vi "NextToken.vi"(8 "error in (no error)":errorcluster, 10 "Index In":i32, 11 "JSON String":string) -> (0 "error out":errorcluster, 1 "TOKEN":T1, 2 "Index Out":i32)   [LabVIEW 2016, in "JSON Value.lvclass"]
uses:
  JSON Value.lvclass
  Token Type.ctl
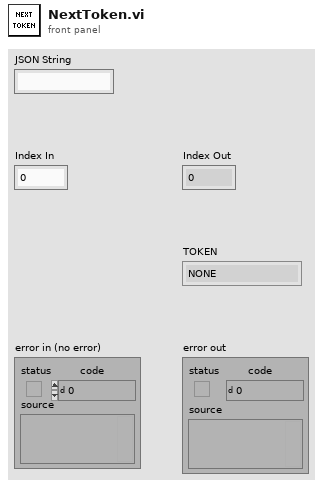
[diagram p1: front panel]
types:
  T1 = typedef "JSON Value.lvclass/Token Type.ctl" = enum8{"NONE", "CURLY_OPEN", "CURLY_CLOSE", "SQUARED_OPEN", "SQUARED_CLOSE", "COLON", "COMMA", "STRING", "NUMBER", "TRUE", "FALSE", "NULL"}
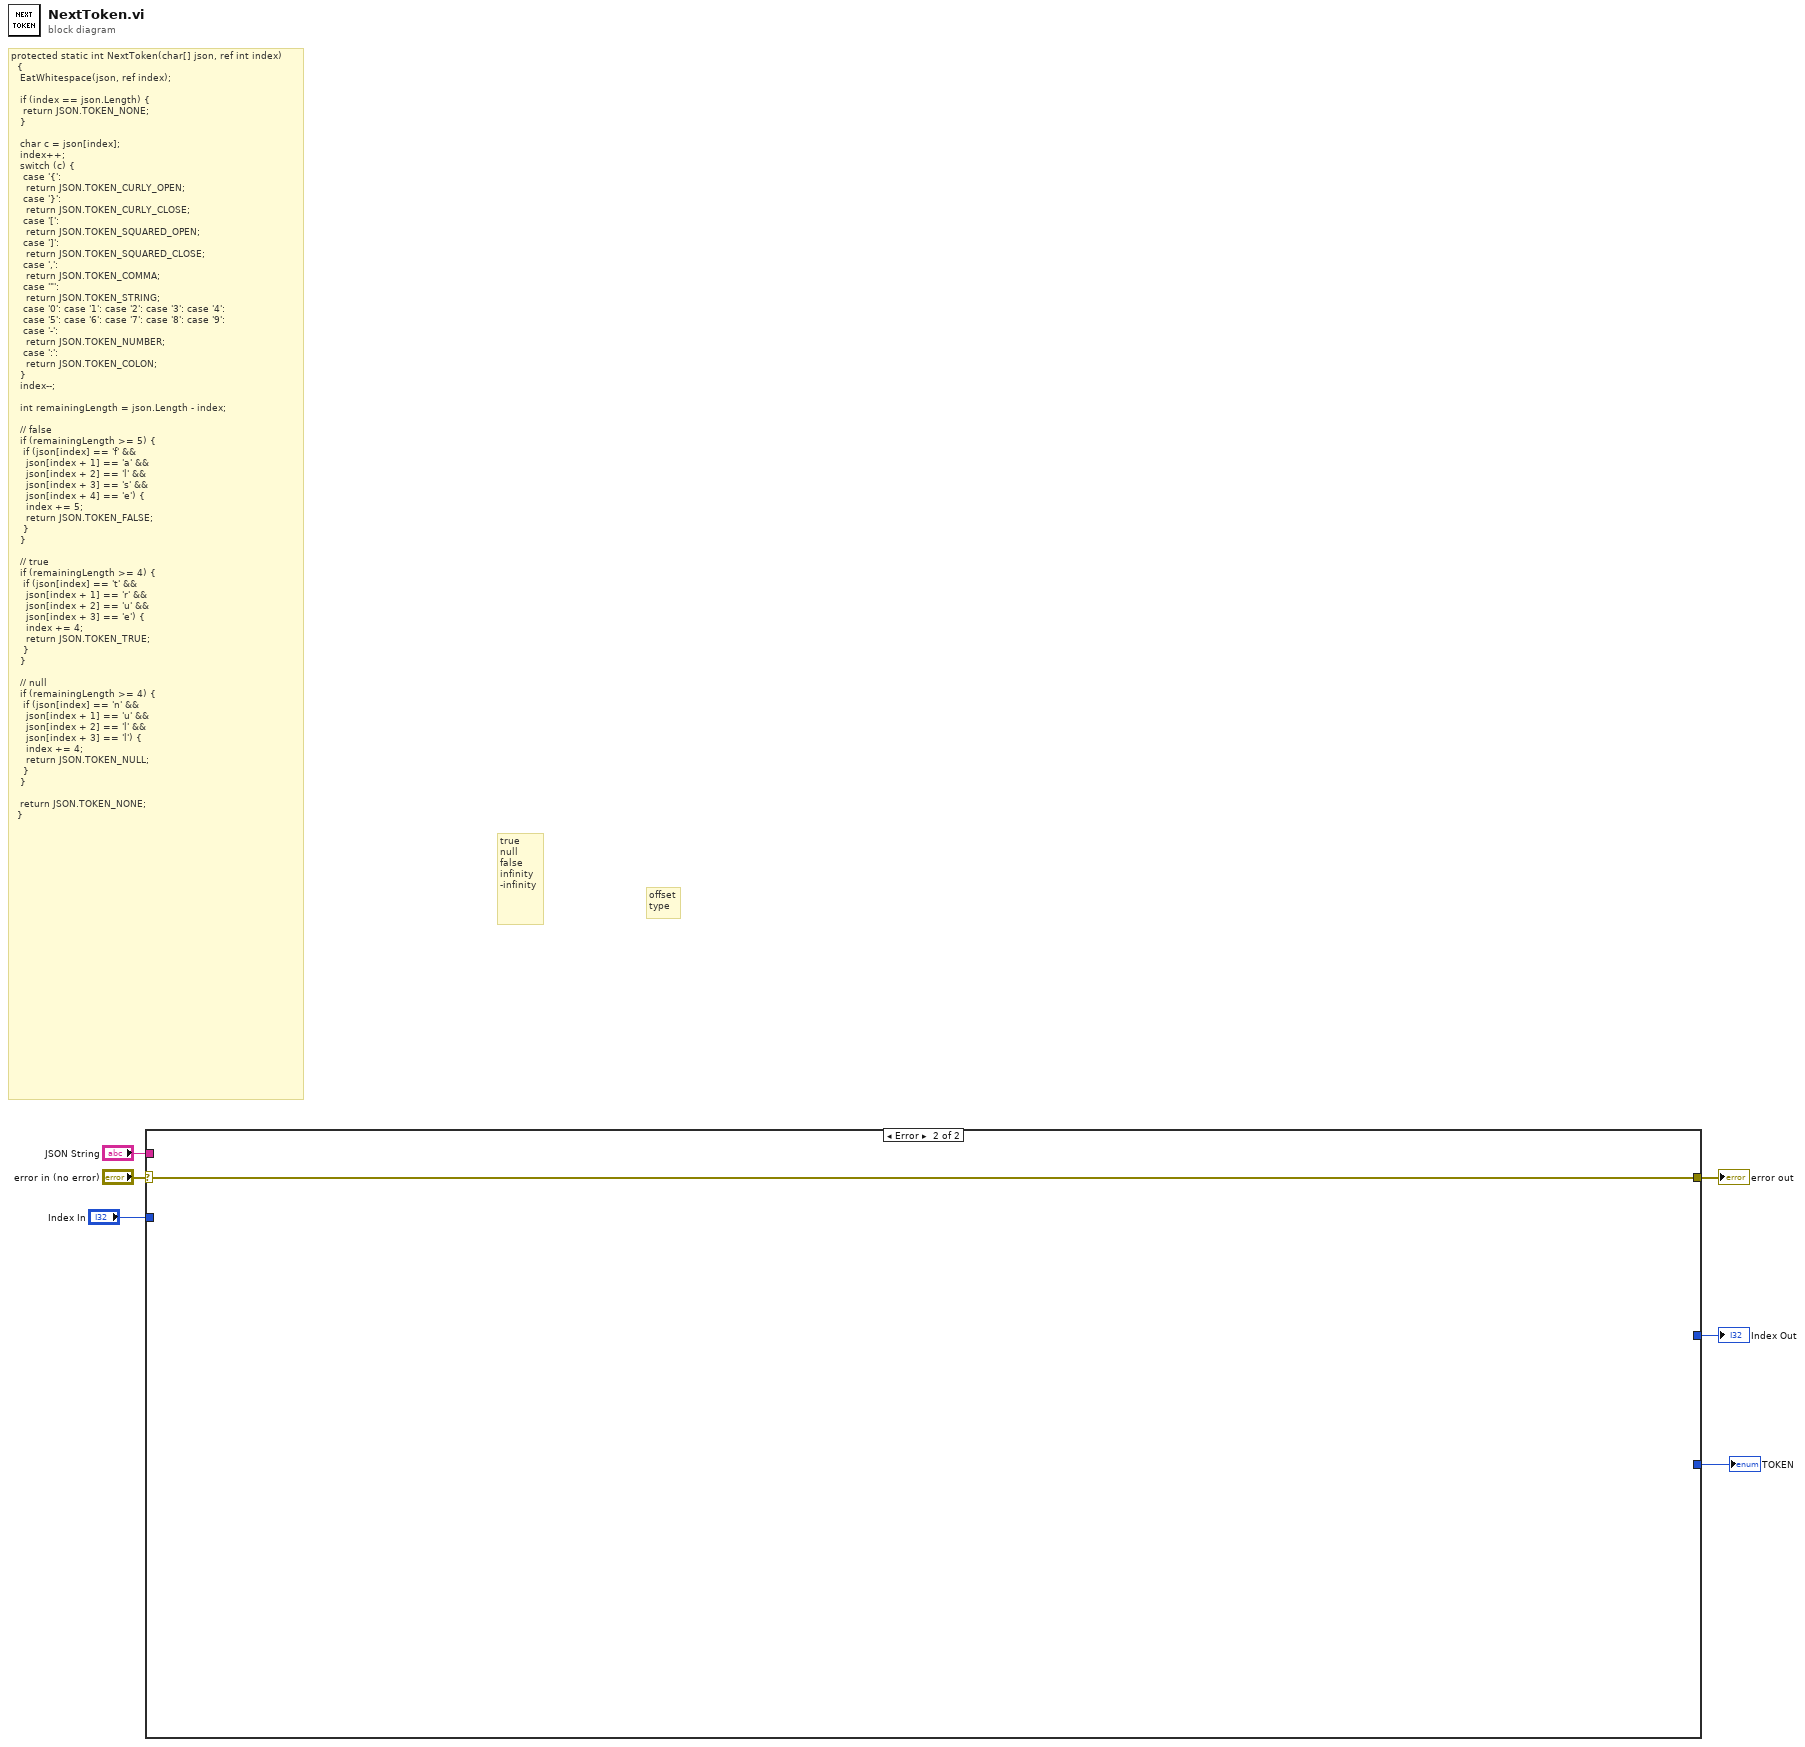
[diagram p0: block diagram]
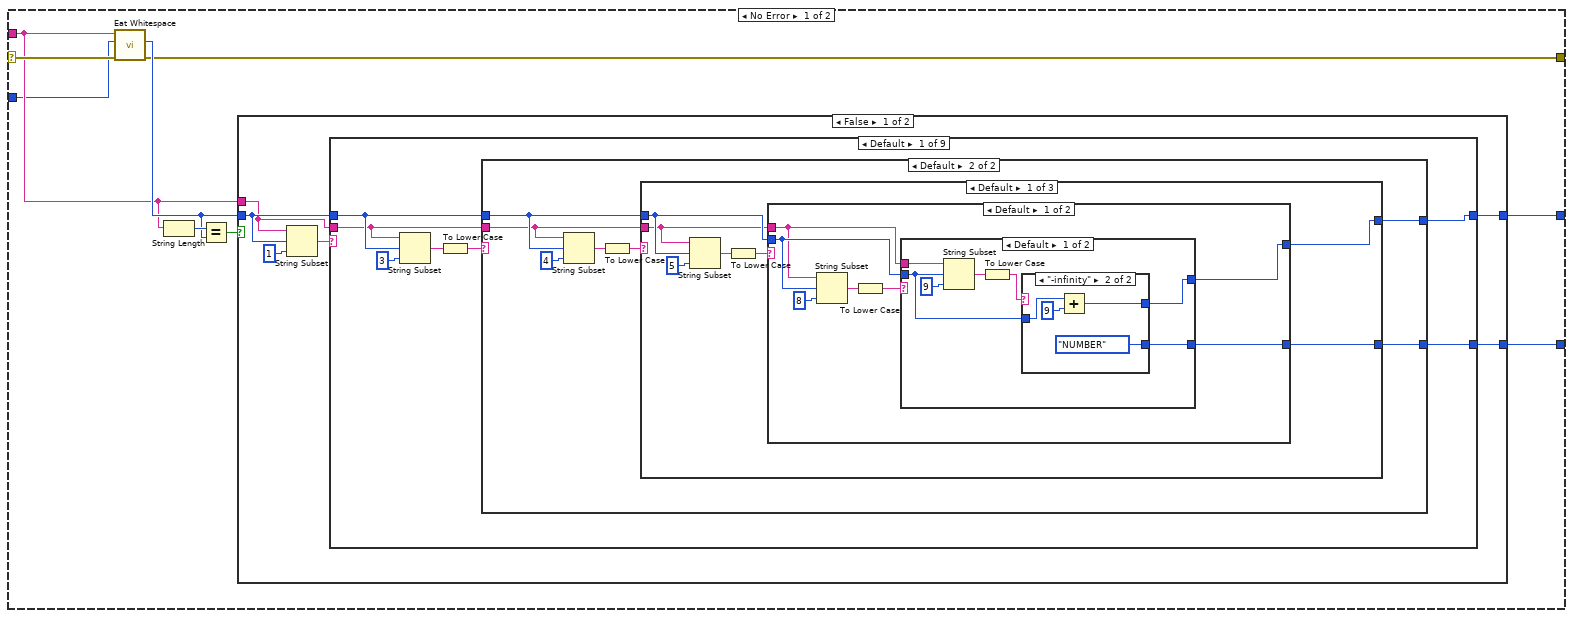
[diagram p2: hidden frame]
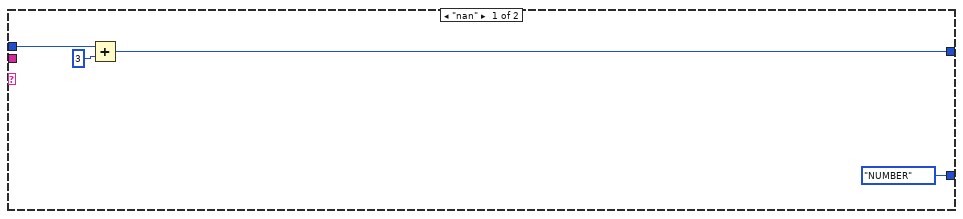
[diagram p3: hidden frame]
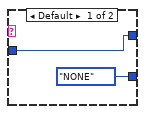
[diagram p4: hidden frame]
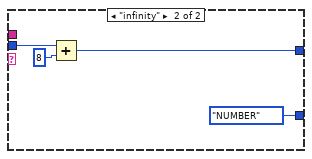
[diagram p5: hidden frame]
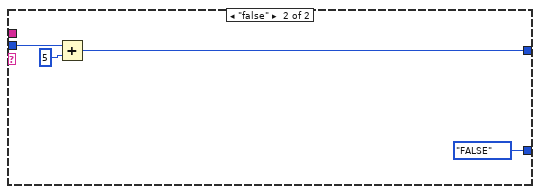
[diagram p6: hidden frame]
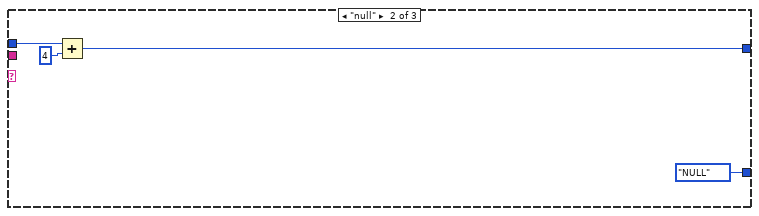
[diagram p7: hidden frame]
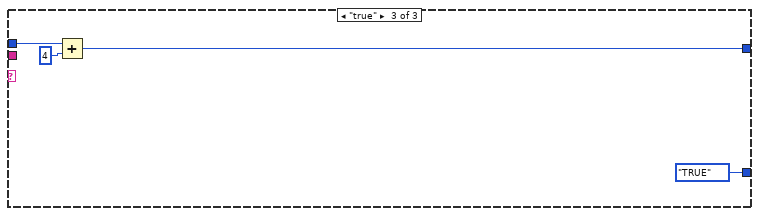
[diagram p8: hidden frame]
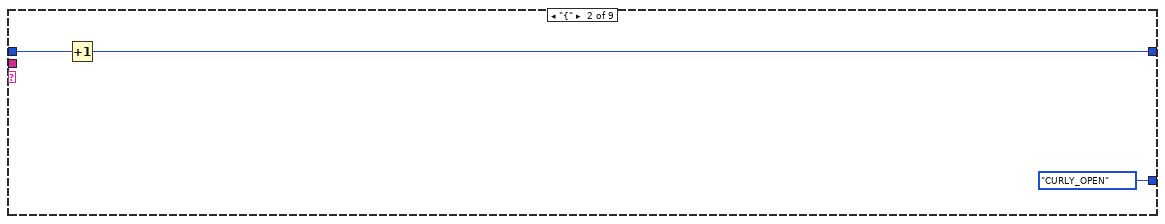
[diagram p9: hidden frame]
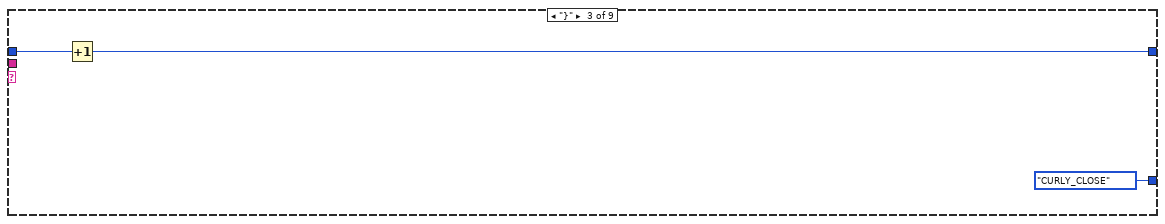
[diagram p10: hidden frame]
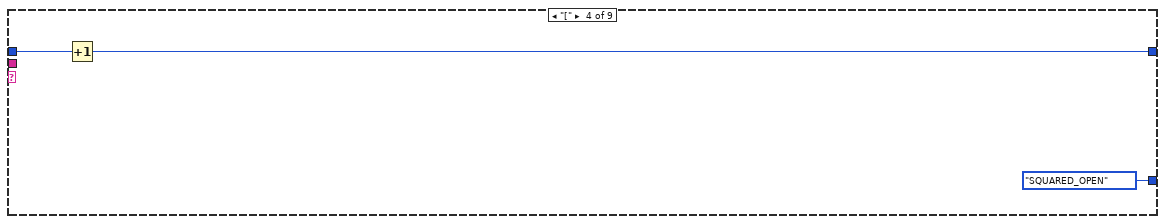
[diagram p11: hidden frame]
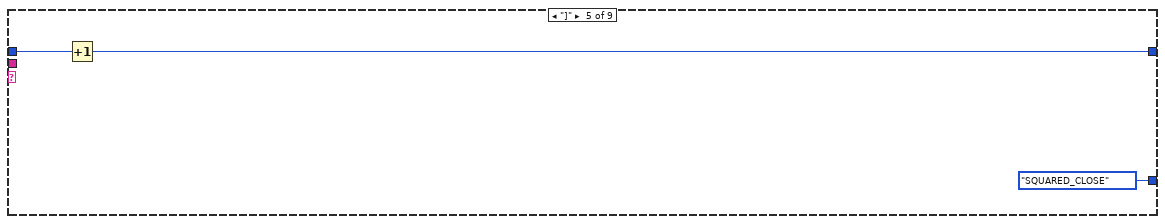
[diagram p12: hidden frame]
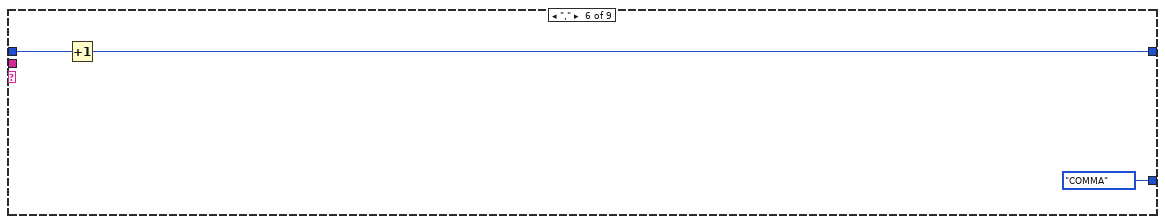
[diagram p13: hidden frame]
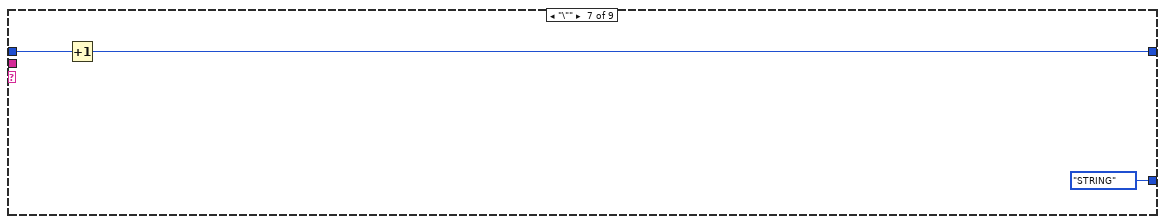
[diagram p14: hidden frame]
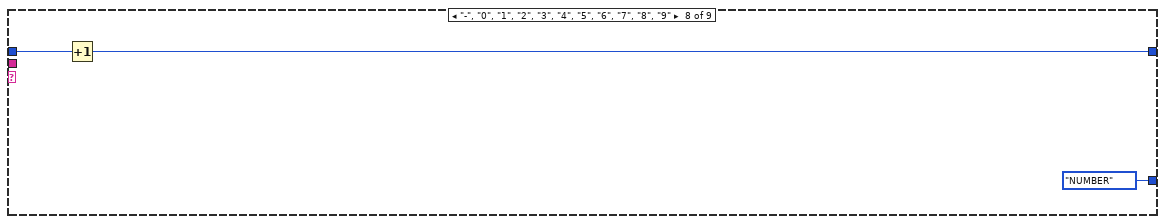
[diagram p15: hidden frame]
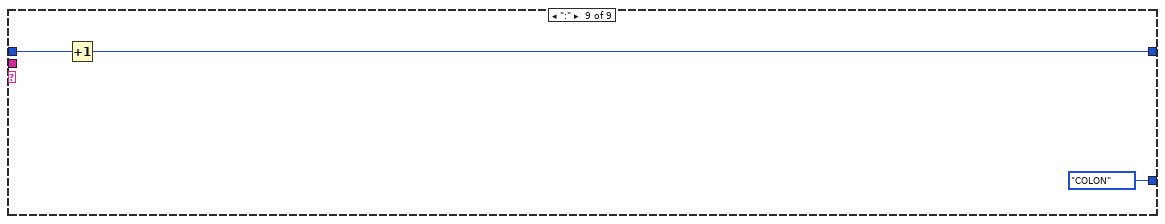
[diagram p16: hidden frame]
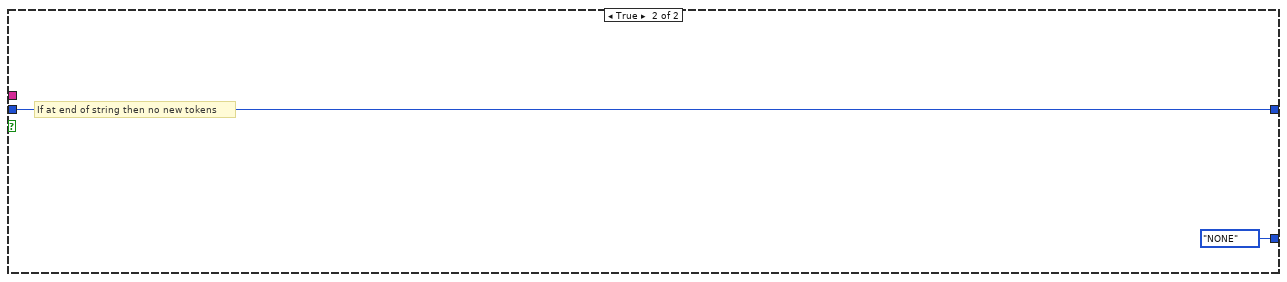
[diagram p17: hidden frame]
diagram:
  # "offset\ntype"
  # "true\nnull\nfalse\ninfinity\n-infinity"
  # "protected static int NextToken(char[] json, ref int index)\n\t\t{\n\t\t\tEatWhitespace(json, ref index);\n\n\t\t\tif (index == json.Length) {\n\t\t\t\treturn JSON.TOKEN_NONE;\n\t\t\t}\n\n\t\t\tchar c = json[index];\n\t\t\tindex++;\n\t\t\tswitch (c) {\n\t\t\t\tcase '{':\n\t\t\t\t\treturn JSON.TOKEN_CURLY_OPEN;\n\t\t\t\tcase '}':\n\t\t\t\t\treturn JSON.TOKEN_CURLY_CLOSE;\n\t\t\t\tcase '[':\n\t\t\t\t\treturn JSON.TOKEN_SQUARED_OPEN;\n\t\t\t\tcase ']':\n\t\t\t\t\treturn JSON.TOKEN_SQUARED_CLOSE;\n\t\t\t\tcase ',':\n\t\t\t\t\treturn JSON.TOKEN_COMMA;\n\t\t\t\tcase '\"':\n\t\t\t\t\treturn JSON.TOKEN_STRING;\n\t\t\t\tcase '0': case '1': case '2': case '3': case '4':\n\t\t\t\tcase '5': case '6': case '7': case '8': case '9':\n\t\t\t\tcase '-':\n\t\t\t\t\treturn JSON.TOKEN_NUMBER;\n\t\t\t\tcase ':':\n\t\t\t\t\treturn JSON.TOKEN_COLON;\n\t\t\t}\n\t\t\tindex--;\n\n\t\t\tint remainingLength = json.Length - index;\n\n\t\t\t// false\n\t\t\tif (remainingLength >= 5) {\n\t\t\t\tif (json[index] == 'f' &&\n\t\t\t\t\tjson[index + 1] == 'a' &&\n\t\t\t\t\tjson[index + 2] == 'l' &&\n\t\t\t\t\tjson[index + 3] == 's' &&\n\t\t\t\t\tjson[index + 4] == 'e') {\n\t\t\t\t\tindex += 5;\n\t\t\t\t\treturn JSON.TOKEN_FALSE;\n\t\t\t\t}\n\t\t\t}\n\n\t\t\t// true\n\t\t\tif (remainingLength >= 4) {\n\t\t\t\tif (json[index] == 't' &&\n\t\t\t\t\tjson[index + 1] == 'r' &&\n\t\t\t\t\tjson[index + 2] == 'u' &&\n\t\t\t\t\tjson[index + 3] == 'e') {\n\t\t\t\t\tindex += 4;\n\t\t\t\t\treturn JSON.TOKEN_TRUE;\n\t\t\t\t}\n\t\t\t}\n\n\t\t\t// null\n\t\t\tif (remainingLength >= 4) {\n\t\t\t\tif (json[index] == 'n' &&\n\t\t\t\t\tjson[index + 1] == 'u' &&\n\t\t\t\t\tjson[index + 2] == 'l' &&\n\t\t\t\t\tjson[index + 3] == 'l') {\n\t\t\t\t\tindex += 4;\n\t\t\t\t\treturn JSON.TOKEN_NULL;\n\t\t\t\t}\n\t\t\t}\n\n\t\t\treturn JSON.TOKEN_NONE;\n\t\t}"
  n1 = case shown="Error" "error in (no error)" {
    selector: "error in (no error)" -> [w15 w109]
    tunnel: [w11 w109] -> w5
    tunnel: "JSON String" -> [w10 _]
    tunnel: "Index In" -> [w9 _]
    tunnel: [w8 _] -> w2
    tunnel: [w7 _] -> w1
    frame No Error {
      n2 = call "Eat Whitespace.vi"("error in (no error)"=w15, "Index In"=w9, "JSON String"=w10) -> ("error out"=w11:errorcluster, "Index Out"=w12:i32)  [unwired: 7 in]
      n3 = String Length(string=w10) -> (length=w14:i32)
      n4 = Equal?(x=w14, y=w12) -> (x = y?=w13:bool)
      n5 = case shown="False" w13 {
        tunnel: [w17 Token_Type."NONE" ("TOKEN")] -> w7
        tunnel: w12 -> [w19 w107]
        tunnel: w10 -> [w16 _]
        tunnel: [w18 w107] -> w8
        frame False {
          n6 = String Subset(string=w16, offset (0)=w19, length (rest)=1 ("length (rest)")) -> (substring=w20:string)
          n7 = case shown="Default" w20 {
            tunnel: w19 -> [w25 w85 w87 w90 w92 w96 w99 w102 w105]
            tunnel: [w24 w84 w86 w89 w93 w95 w98 w101 w104] -> w18
            tunnel: [w23 Token_Type."CURLY_OPEN" ("TOKEN") Token_Type."CURLY_CLOSE" ("TOKEN") Token_Type."SQUARED_OPEN" ("TOKEN") Token_Type."SQUARED_CLOSE" ("TOKEN") Token_Type."COMMA" ("TOKEN") Token_Type."STRING" ("TOKEN") Token_Type."NUMBER" ("TOKEN") Token_Type."COLON" ("TOKEN")] -> w17
            tunnel: w16 -> [w22 _ _ _ _ _ _ _ _]
            frame Default {
              n8 = String Subset(string=w22, offset (0)=w25, length (rest)=3 ("length (rest)")) -> (substring=w27:string)
              n9 = To Lower Case(string=w27) -> (all lower case string=w26:string)
              n10 = case shown="Default" w26 {
                tunnel: w25 -> [w32 w36]
                tunnel: [w31 w35] -> w24
                tunnel: [Token_Type."NUMBER" ("TOKEN") w34] -> w23
                tunnel: w22 -> [_ w33]
                frame "nan" {
                  n11 = Add(x=w32, y=3) -> (x+y=w31:i32)
                }
                frame Default {
                  n12 = String Subset(string=w33, offset (0)=w36, length (rest)=4 ("length (rest)")) -> (substring=w39:string)
                  n13 = To Lower Case(string=w39) -> (all lower case string=w37:string)
                  n14 = case shown="Default" w37 {
                    tunnel: w36 -> [w41 w78 w82]
                    tunnel: [w42 w76 w80] -> w35
                    tunnel: [w43 Token_Type."NULL" ("TOKEN") Token_Type."TRUE" ("TOKEN")] -> w34
                    tunnel: w33 -> [w40 _ _]
                    frame Default {
                      n15 = String Subset(string=w40, offset (0)=w41, length (rest)=5 ("length (rest)")) -> (substring=w45:string)
                      n16 = To Lower Case(string=w45) -> (all lower case string=w44:string)
                      n17 = case shown="Default" w44 {
                        tunnel: w41 -> [w50 w74]
                        tunnel: [w48 w72] -> w42
                        tunnel: [w49 Token_Type."FALSE" ("TOKEN")] -> w43
                        tunnel: w40 -> [w47 _]
                        frame Default {
                          n18 = String Subset(string=w47, offset (0)=w50, length (rest)=8 ("length (rest)")) -> (substring=w52:string)
                          n19 = To Lower Case(string=w52) -> (all lower case string=w53:string)
                          n20 = case shown="Default" w53 {
                            tunnel: w50 -> [w56 w70]
                            tunnel: [w55 w68] -> w48
                            tunnel: [w54 Token_Type."NUMBER" ("TOKEN")] -> w49
                            tunnel: w47 -> [w57 _]
                            frame Default {
                              n21 = String Subset(string=w57, offset (0)=w56, length (rest)=9 ("length (rest)")) -> (substring=w59:string)
                              n22 = To Lower Case(string=w59) -> (all lower case string=w60:string)
                              n23 = case shown="\"-infinity\"" w60 {
                                tunnel: w56 -> [w61 w66]
                                tunnel: [w61 w64] -> w55
                                tunnel: [Token_Type."NONE" ("TOKEN") Token_Type."NUMBER" ("TOKEN")] -> w54
                                frame Default {
                                }
                                frame "-infinity" {
                                n24 = Add(x=w66, y=9) -> (x+y=w64:i32)
                                }
                              }
                            }
                            frame "infinity" {
                              n25 = Add(x=w70, y=8) -> (x+y=w68:i32)
                            }
                          }
                        }
                        frame "false" {
                          n26 = Add(x=w74, y=5) -> (x+y=w72:i32)
                        }
                      }
                    }
                    frame "null" {
                      n27 = Add(x=w78, y=4) -> (x+y=w76:i32)
                    }
                    frame "true" {
                      n28 = Add(x=w82, y=4) -> (x+y=w80:i32)
                    }
                  }
                }
              }
            }
            frame "{" {
              n29 = Increment(x=w85) -> (x+1=w84:i32)
            }
            frame "}" {
              n30 = Increment(x=w87) -> (x+1=w86:i32)
            }
            frame "[" {
              n31 = Increment(x=w90) -> (x+1=w89:i32)
            }
            frame "]" {
              n32 = Increment(x=w92) -> (x+1=w93:i32)
            }
            frame "," {
              n33 = Increment(x=w96) -> (x+1=w95:i32)
            }
            frame "\"" {
              n34 = Increment(x=w99) -> (x+1=w98:i32)
            }
            frame "-", "0", "1", "2", "3", "4", "5", "6", "7", "8", "9" {
              n35 = Increment(x=w102) -> (x+1=w101:i32)
            }
            frame ":" {
              n36 = Increment(x=w105) -> (x+1=w104:i32)
            }
          }
        }
        frame True {
          # "If at end of string then no new tokens"
        }
      }
    }
    frame Error {
    }
  }
  "error out" <- w5
  "Index Out" <- w2
  "TOKEN" <- w1
